vi "Find-Path-with-Astar.vi"(8 "error in (no error)":errorcluster, 9 "goal node":cluster{"X":i32, "Y":i32}={"X"=32, "Y"=32}, 10 "start node":cluster{"X":i32, "Y":i32}={"X"=3, "Y"=3}, 11 "map reference in":refnum<data-value>) -> (0 "error out":errorcluster, 1 "Array":cluster{"X":i32, "Y":i32}[](array[cluster]), 3 "map reference out":refnum<data-value>)   [LabVIEW 2017]
uses:
  <vilib>/robotics/Navigation/shared/WorldMap/OccupancyGridWorldMap/NI_Robotics_OccupancyGridWorldMap.lvclass
  C:/Program Files (x86)/National Instruments/LabVIEW 2017/vi.lib/robotics/Navigation/shared/WorldMap/AbstractWorldMap/NI_Robotics_AbstractWorldMap.lvclass
  <vilib>/robotics/Navigation/shared/MapNode/OccupancyGridNode/NI_Robotics_OccupancyGridMapNode.lvclass
  C:/Program Files (x86)/National Instruments/LabVIEW 2017/vi.lib/robotics/Navigation/shared/MapNode/AbstractAstarNode/NI_Robotics_AbstractAstarNode.lvclass
  <vilib>/robotics/Navigation/NI_Robotics_Navigation .lvlib
panel:
  out "intensity values":dbl[][](array[numeric])
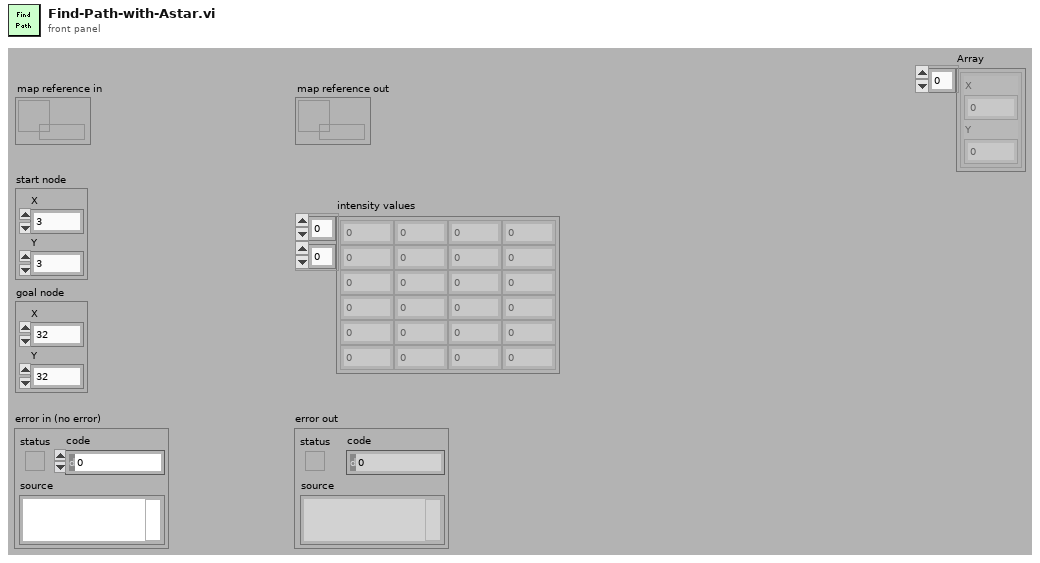
[diagram p1: front panel]
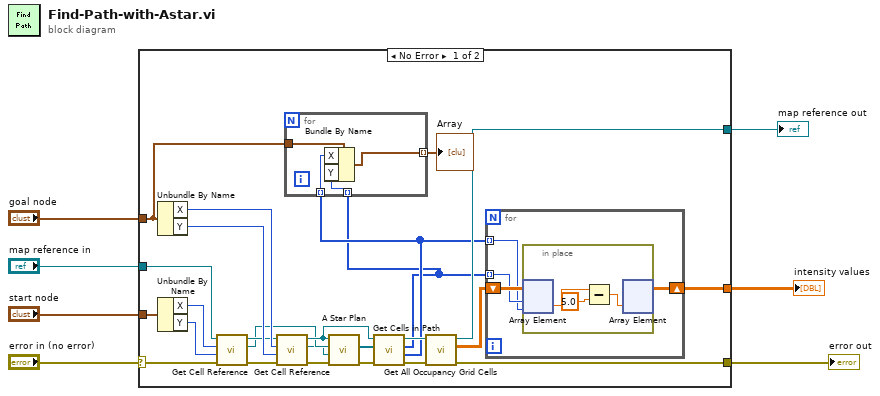
[diagram p0: block diagram]
diagram:
  n1 = case shown="No Error" "error in (no error)" {
    selector: "error in (no error)" -> [w16 w44]
    tunnel: "map reference in" -> [w17 w45]
    tunnel: "goal node" -> [w11 _]
    tunnel: "start node" -> [w15 _]
    tunnel: [w14 _] -> w3
    tunnel: [w13 w45] -> w2
    tunnel: [w12 w44] -> w1
    frame No Error {
      n2 = Unbundle By Name(w11) -> ("X"=w31:i32, "Y"=w32:i32)
      n3 = Unbundle By Name(w15) -> ("X"=w29:i32, "Y"=w30:i32)
      n4 = call <vilib>:"Get Cell Reference.vi"("error in (no error)"=w16, "y"=w30, "x"=w29, "map reference in"=w17) -> ("error out"=w21:errorcluster, "cell reference"=w19:refnum<data-value>, "map reference out"=w25:refnum<data-value>)  [unwired: 4 in, 1 out]
      n5 = call <vilib>:"Get Cell Reference.vi"("error in (no error)"=w21, "y"=w32, "x"=w31, "map reference in"=w25) -> ("error out"=w26:errorcluster, "cell reference"=w18:refnum<data-value>, "map reference out"=w23:refnum<data-value>)  [unwired: 4 in, 1 out]
      n6 = call <vilib>:"A Star Plan.vi"("error in (no error)"=w26, "goal reference"=w18, "start reference"=w19, "map reference in"=w23) -> ("error out"=w27:errorcluster, "path references"=w24:refnum<data-value>[])  [unwired: 4 in, 2 out]
      n7 = call <vilib>:"Get Cells in Path.vi"("error in (no error)"=w27, "path references"=w24, "map reference in"=w23) -> ("error out"=w20:errorcluster, "y coordinates"=w10:i32[], "x coordinates"=w9:i32[], "map reference out"=w22:refnum<data-value>)  [unwired: 5 in]
      n8 = for {
        tunnel: w11 -> [w36]
        tunnel: w10 -> [w35] mode=indexing
        tunnel: w9 -> [w34] mode=indexing
        tunnel: [w33] -> w8 mode=indexing
        n9 = Bundle By Name(cluster=w36, "X"=w35, "Y"=w34) -> (w33:cluster{"X":i32, "Y":i32})
      }
      "Array" <- w8
      n10 = call <vilib>:"Get All Occupancy Grid Cells.vi"("error in (no error)"=w20, "map reference in"=w22) -> ("error out"=w12:errorcluster, "occupancy grid"=w28:dbl[][], "map reference out"=w13:refnum<data-value>)  [unwired: 7 in]
      n11 = for {
        tunnel: w10 -> [w38] mode=indexing
        tunnel: w9 -> [w39] mode=indexing
        shift-right: [w37] -> w14
        shift-left: w28 -> [w40]
        n12 = in-place {
          n13 = in-place-array #1(w40, w39, w38) -> (w42:dbl)
          n14 = Subtract(x=w42, y=5.0) -> (x-y=w41:dbl)
          n15 = in-place-array #1(w41) -> (w37:dbl[][])  [unwired: 2 out]
        }
      }
    }
    frame Error {
    }
  }
  "error out" <- w1
  "intensity values" <- w3
  "map reference out" <- w2
